vi "Set Values by Primary Key.vi"(8 "error in (no error)":errorcluster, 10 "Primary Key Value":string, 11 "Table in":refnum<class "Basic Table.lvclass">) -> (0 "error out":errorcluster, 3 "Table out":refnum<class "Basic Table.lvclass">)   [LabVIEW 2020, in "Table.lvlib" / "Basic Table.lvclass"]
uses:
  Basic Table.lvclass
  Basic Table.lvclass/Basic Table.ctl
  Table Configuration Interface/Table Configuration Interface.lvclass
  Column Libraries/Column Interface/Column Interface Class/Column Interface.lvclass
  Database Libraries/Database Interfaces/Database Interface Class/Database Interface.lvclass
panel:
  # "Use this VI to set the value of ALL columns in a table by PK.\nTo set individual columns, use column PK methods."
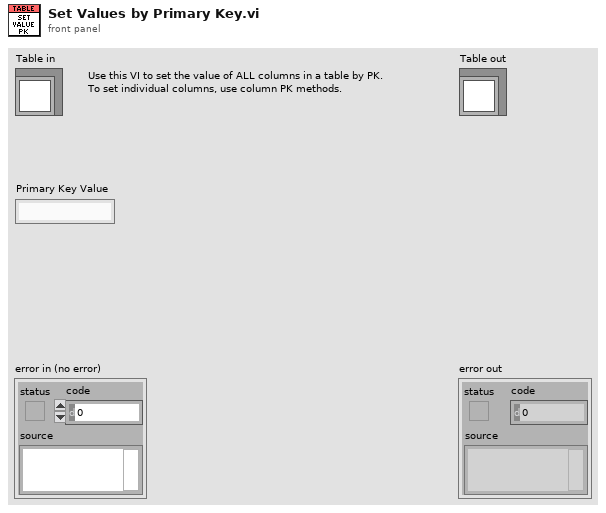
[diagram p1: front panel]
types:
  T1 = map{string, refnum<class "Column Interface.lvclass">}
  T2 = typedef "Database Interfaces.lvlib/Primary Key Info.ctl" = cluster{"Primary Key Column":string, "Display Column":string}
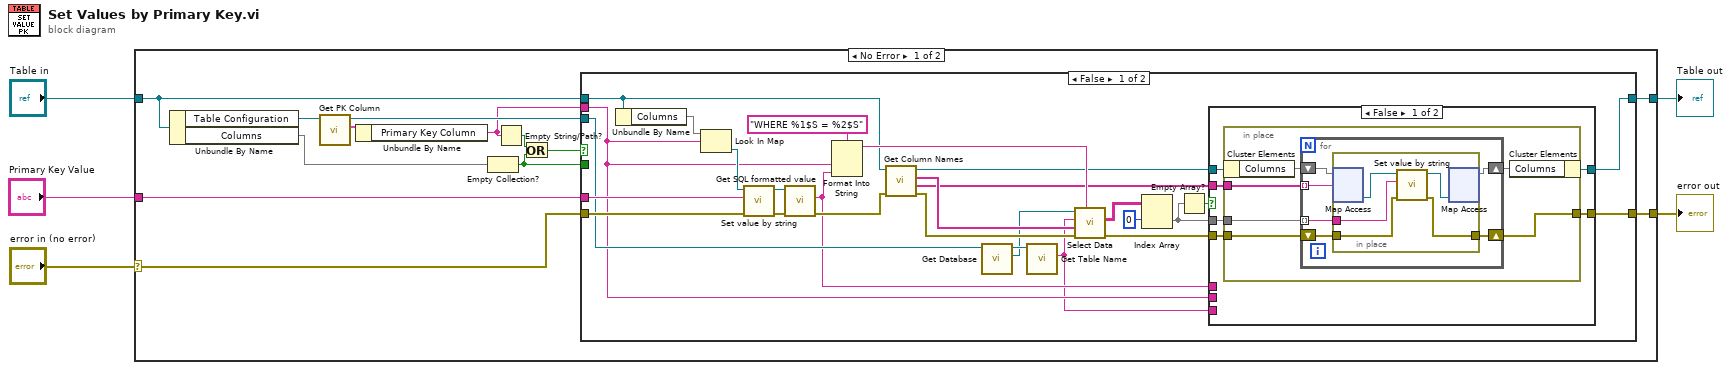
[diagram p0: block diagram]
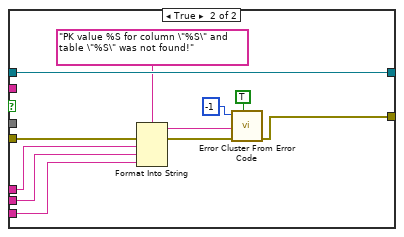
[diagram p2: hidden frame]
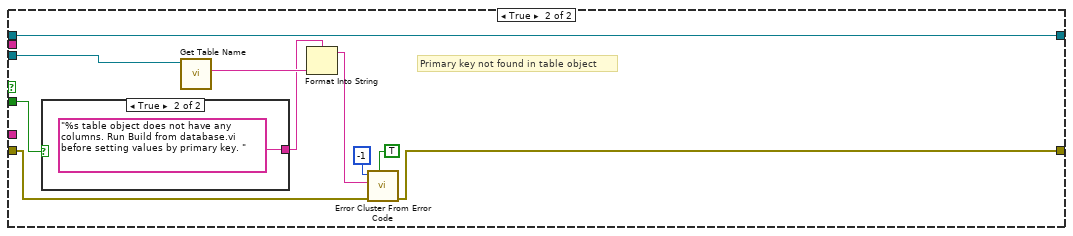
[diagram p3: hidden frame]
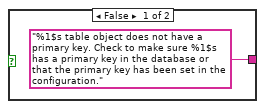
[diagram p4: hidden frame]
diagram:
  n1 = case shown="No Error" "error in (no error)" {
    selector: "error in (no error)" -> [w15 w93]
    tunnel: [w14 w93] -> w4
    tunnel: [w10 w92] -> w2
    tunnel: "Table in" -> [w11 w92]
    tunnel: "Primary Key Value" -> [w18 _]
    frame No Error {
      n2 = Unbundle By Name(w11) -> ("Table Configuration"=w9:refnum<class "Table Configuration Interface.lvclass">, "Columns"=w17:T1)
      n3 = call-dynamic "Get PK Column.vi"("Table Configuration Interface in"=w9) -> ("Primary Key"=w7:T2, "Table Configuration Interface out"=w8:refnum<class "Table Configuration Interface.lvclass">)  [unwired: 8 in, 1 out]
      n4 = Unbundle By Name(w7) -> ("Primary Key Column"=w6:string)
      n5 = Empty Collection?(1:w17) -> (0:w13:bool)
      n6 = Empty String/Path?(string/path=w6) -> (empty?=w12:bool)
      n7 = Or(x=w12, y=w13) -> (x .or. y?=w16:bool)
      n8 = case shown="False" w16 {
        tunnel: w18 -> [w37 _]
        tunnel: w6 -> [w21 _]
        tunnel: w15 -> [w36 w86]
        tunnel: [w39 w85] -> w14
        tunnel: w13 -> [_ w89]
        tunnel: w11 -> [w27 w84]
        tunnel: [w28 w84] -> w10
        tunnel: w8 -> [w26 w82]
        frame False {
          n9 = Unbundle By Name(w27) -> ("Columns"=w43:T1)
          n10 = Look In Map(map=w43, key=w21) -> (value=w38:refnum<class "Column Interface.lvclass">)  [unwired: 1 in, 1 out]
          n11 = call-dynamic "Set value by string.vi"("error in (no error)"=w36, "Value"=w37, "Column Interface in"=w38) -> ("error out"=w34:errorcluster, "Column Interface out"=w35:refnum<class "Column Interface.lvclass">)  [unwired: 7 in]
          n12 = call-dynamic "Get SQL formatted value.vi"("error in (no error)"=w34, "Column Interface in"=w35) -> ("error out"=w33:errorcluster, "Formatted Value"=w20:string)  [unwired: 7 in, 1 out]
          n13 = Format Into String(format string="WHERE %1$S = %2$S", w21, w20) -> (resulting string=w44:string)  [unwired: 2 in, 1 out]
          n14 = call "Get Column Names.vi"("error in (no error)"=w33, "Table in"=w27) -> ("error out"=w32:errorcluster, "Key Names"=w30:string[], "Column Names"=w31:string[], "Table out"=w29:refnum<class "Basic Table.lvclass">)  [unwired: 6 in]
          n15 = call-dynamic "Get Database.vi"("Table Configuration Interface in"=w26) -> ("Database"=w24:refnum<class "Database Interface.lvclass">, "Table Configuration Interface out"=w25:refnum<class "Table Configuration Interface.lvclass">)  [unwired: 8 in, 1 out]
          n16 = call-dynamic "Get Table Name.vi"("Table Configuration Interface in"=w25) -> ("Table Name"=w19:string)  [unwired: 8 in, 2 out]
          n17 = call-dynamic "Select Data.vi"("WHERE Statement"=w44, "error in (no error)"=w32, "Columns"=w31, "Table"=w19, "Database Interface in"=w24) -> ("error out"=w40:errorcluster, "Data"=w42:string[][])  [unwired: 4 in, 1 out]
          n18 = Index Array(array=w42, index (row)=0) -> (element=w22:string[])  [unwired: 1 in]
          n19 = Empty Array?(array=w22) -> (empty?=w23:bool)
          n20 = case shown="False" w23 {
            tunnel: w40 -> [w51 w77]
            tunnel: [w50 w69] -> w39
            tunnel: w30 -> [w49 _]
            tunnel: w29 -> [w48 w79]
            tunnel: [w47 w79] -> w28
            tunnel: w22 -> [w46 _]
            tunnel: w21 -> [_ w75]
            tunnel: w20 -> [_ w76]
            tunnel: w19 -> [_ w74]
            frame False {
              n21 = in-place {
                in-place-border: w51 -> [w57]
                in-place-border: [w56] -> w50
                in-place-border: w49 -> [w55]
                in-place-border: w46 -> [w52]
                n22 = in-place-cluster #1(w48) -> ("Columns"=w54:T1)
                n23 = for {
                  tunnel: w55 -> [w63] mode=indexing
                  shift-right: [w61] -> w53
                  shift-left: w54 -> [w62]
                  shift-right: [w59] -> w56
                  shift-left: w57 -> [w60]
                  tunnel: w52 -> [w58] mode=indexing
                  n24 = in-place {
                    in-place-border: w60 -> [w66]
                    in-place-border: [w65] -> w59
                    in-place-border: w58 -> [w64]
                    n25 = in-place-map #2(w62, w63) -> (w68:refnum<class "Column Interface.lvclass">)  [unwired: 1 in, 1 out]
                    n26 = call-dynamic "Set value by string.vi"("error in (no error)"=w66, "Value"=w64, "Column Interface in"=w68) -> ("error out"=w65:errorcluster, "Column Interface out"=w67:refnum<class "Column Interface.lvclass">)  [unwired: 7 in]
                    n27 = in-place-map #2(w67) -> (w61:T1)  [unwired: 1 in, 2 out]
                  }
                }
                n28 = in-place-cluster #1("Columns"=w53) -> (w47:refnum<class "Basic Table.lvclass">)
              }
            }
            frame True {
              n29 = Format Into String(format string="PK value %S for column \"%S\" and table \"%S\" was not found!", error in=w77, w76, w75, w74) -> (resulting string=w73:string, error out=w70:errorcluster)  [unwired: 1 in]
              n30 = call <vilib>:"Error Cluster From Error Code.vi"("show call chain? (False)"=TRUE, "error in (no error)"=w70, "error message (\"\")"=w73, "error code (0)"=-1) -> ("error out"=w69:errorcluster)  [unwired: 5 in]
            }
          }
        }
        frame True {
          # "Primary key not found in table object"
          n31 = case shown="True" w89 {
            tunnel: ["%1$s table object does not have a primary key. Check to make sure %1$s has a primary key in the database or that the primary key has been set in the configuration." "%s table object does not have any columns. Run Build from database.vi before setting values by primary key. "] -> w80
            frame False {
            }
            frame True {
            }
          }
          n32 = call-dynamic "Get Table Name.vi"("Table Configuration Interface in"=w82) -> ("Table Name"=w83:string)  [unwired: 8 in, 2 out]
          n33 = Format Into String(format string=w80, w83) -> (resulting string=w81:string)  [unwired: 2 in, 1 out]
          n34 = call <vilib>:"Error Cluster From Error Code.vi"("show call chain? (False)"=TRUE, "error in (no error)"=w86, "error message (\"\")"=w81, "error code (0)"=-1) -> ("error out"=w85:errorcluster)  [unwired: 5 in]
        }
      }
    }
    frame Error {
    }
  }
  "error out" <- w4
  "Table out" <- w2
